vi "Set Delay.vi"(6 "Delay (s)":dbl min=0.0 max=999.999 step=5e-11, 8 "error in (no error)":errorcluster, 9 "Sync To":T1, 10 "Channel":T1, 11 "VISA Refnum in":refnum<visa-resource-name>) -> (0 "error out":errorcluster)   [LabVIEW 2012, in "SRS_DG535_Lib.lvlib"]
uses:
  SRS_DG535_Lib.lvlib
  Command/DG535_Channel.ctl
panel:
  out "resulting string":string
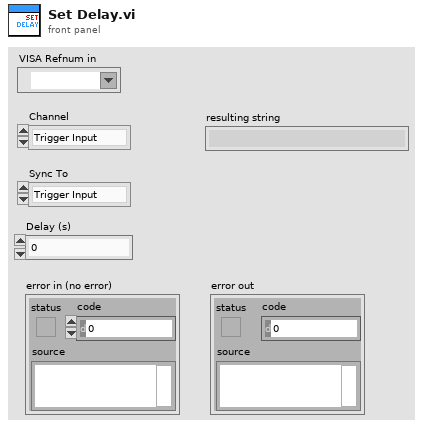
[diagram p1: front panel]
types:
  T1 = typedef "SRS_DG535_Lib.lvlib/DG535_Channel.ctl" = enum16{"Trigger Input", "T0 Output", "A Output", "B Output", "AB Output", "C Output", "D Output", "CD Output", "NULL"}
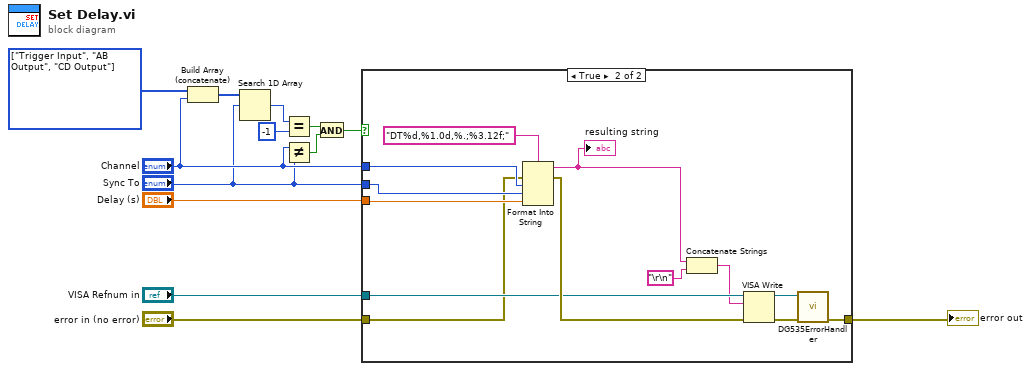
[diagram p0: block diagram]
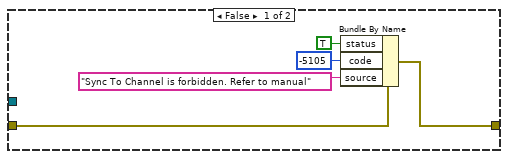
[diagram p2: hidden frame]
diagram:
  w11 = T1[] [enum."Trigger Input", enum."AB Output", enum."CD Output"] items=["Trigger Input", "T0 Output", "A Output", "B Output", "AB Output", "C Output", "D Output", "CD Output", "NULL"]
  n1 = Build Array (concatenate)(w11, "Channel") -> (w10:T1[])
  n2 = Search 1D Array(1D array=w10, element="Sync To") -> (index of element=w8:i32)  [unwired: 1 in]
  n3 = Equal?(x=w8, y=-1) -> (x = y?=w5:bool)
  n4 = Not Equal?(x="Channel", y="Sync To") -> (x != y?=w1:bool)
  n5 = And(x=w5, y=w1) -> (x .and. y?=w2:bool)
  n6 = case shown="True" w2 {
    tunnel: "Delay (s)" -> [_ w31]
    tunnel: [w17 w19] -> w6
    tunnel: "VISA Refnum in" -> [_ w27]
    tunnel: "Channel" -> [_ w24]
    tunnel: "Sync To" -> [_ w23]
    tunnel: "error in (no error)" -> [w18 w22]
    frame False {
      n7 = Bundle By Name(cluster=w18, "status"=TRUE, "code"=-5105, "source"="Sync To Channel is forbidden. Refer to manual") -> (w17:errorcluster)
    }
    frame True {
      n8 = Format Into String(format string="DT%d,%1.0d,%.;%3.12f;", error in=w22, w24, w23, w31) -> (resulting string=w26:string, error out=w29:errorcluster)  [unwired: 1 in]
      "resulting string" <- w26
      n9 = Concatenate Strings(w26, "\r\n") -> (w25:string)
      n10 = VISA Write(VISA resource name=w27, write buffer=w25, error in (no error)=w29) -> (VISA resource name out=w20:refnum<visa-resource-name>, error out=w21:errorcluster)  [unwired: 1 out]
      n11 = call "DG535ErrorHandler.vi"("error in"=w21, "VISA resource name"=w20) -> ("error out"=w19:errorcluster)  [unwired: 7 in, 2 out]
    }
  }
  "error out" <- w6
